vi "ROI entry-Set Z-stack folder path ctrl.vi"(8 "error in (no error)":errorcluster, 11 "Experiment folder path OR Z-stack images folder path":path) -> (0 "error out":errorcluster)   [LabVIEW 2020]
uses:
  ROI Entry screen/Globals/gl_ROI Entry UI globals.vi
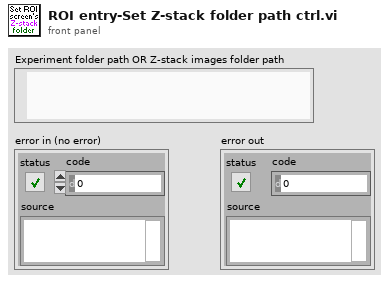
[diagram p1: front panel]
types:
  T1 = typedef "Fixed strings.ctl" = cluster{"ROI file name":string, "Normalised ROI file name":string, "Zplane Pockels values file name":string, "Functional data folder name":string, "Experiment Header file name":string, "Z-stack images folder name":string, "Groups setup rel. path":string, "Groups text file rel. path":string, "TDMS files folder name (F.img)":string, "TDMS files folder name (V.acq)":string, "TDMS files folder name (Pl.acq)":string, "Cycle rel times sequence file":string, "Dynamically called VIs folder name":string, "Time Series folder base name":string}
  T2 = typedef "ROI entry screen ctrl refs cluster.ctl" = cluster{"Done button":refnum<vi>, "Imaging button":refnum<vi>, "Acquisition button":refnum<vi>, "Scan dwell time per pixel (us)":refnum<vi>, "# of planes":refnum<vi>, "Zoom Ctrl":refnum<vi>, "Equal size":refnum<vi>, "Channel":refnum<vi>, "Image Display":refnum<vi>, "Z-Plane Selector":refnum<vi>, "Number of lines left":refnum<vi>, "Z-stack folder path":refnum<vi>, "POI Density":refnum<vi>, "Arb Plane Entry":refnum<vi>, "Whole Plane":refnum<vi>, "Line Mode":refnum<vi>, "Clear Last":refnum<vi>, "Clear All":refnum<vi>, "Delete Lines":refnum<vi>, "Trial Length (sec)":refnum<vi>, "Palette Type":refnum<vi>, "Intensity slider":refnum<vi>, "# POI":refnum<vi>, "Max Z Proj":refnum<vi>, "Zplane ind":refnum<vi>, "Wavelength (nm)":refnum<vi>, "Number of Trials":refnum<vi>, "Funct stim.trig.enable":refnum<vi>, "Funct stim.trig.delay (s)":refnum<vi>, "Line Mode":refnum<vi>, "Step size (µm)":refnum<vi>, "ROI move mode":refnum<vi>, "Cool-down time (s)":refnum<vi>, "Enable cool-down time":refnum<vi>, "Motor Z ind. (um)":refnum<vi>, "AOL Z ind. (um)":refnum<vi>, "Load Reference Image":refnum<vi>, "Rel.  Res.":refnum<vi>, "ROI LIST":refnum<vi>, "Show All":refnum<vi>, "ROI Type":refnum<vi>, "Start Plane":refnum<vi>, "Stop Plane":refnum<vi>, "Offset ROI":refnum<vi>, "Tab Control":refnum<vi>, "Laser Power(%)":refnum<vi>, "Cycle rate":refnum<vi>, "FOV (Ind.)":refnum<vi>, "Frame Size (Ind.)":refnum<vi>, "Resolution (Ind.)":refnum<vi>, "Pixel Density (Ind)":refnum<vi>, "Laser Power (Ind.)":refnum<vi>, "Dwell Time (Ind.)":refnum<vi>, "Adj MC":refnum<vi>}
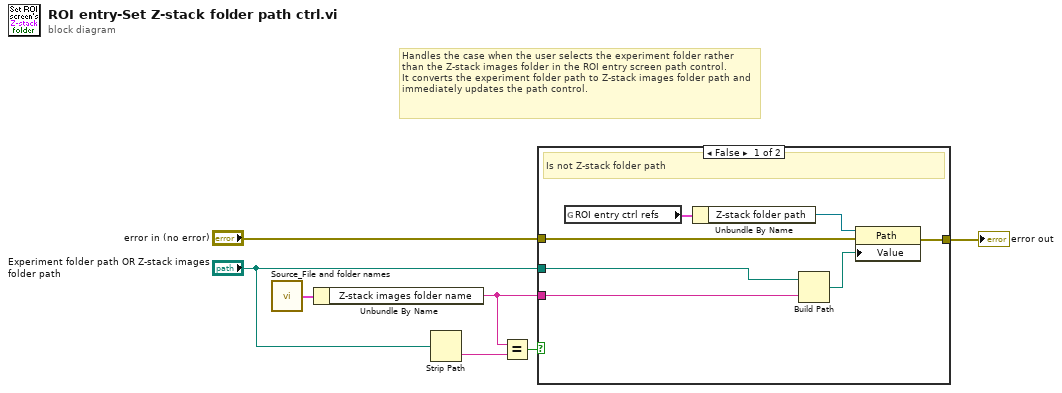
[diagram p0: block diagram]
diagram:
  # "Handles the case when the user selects the experiment folder rather than the Z-stack images folder in the ROI entry screen path control.\nIt converts the experiment folder path to Z-stack images folder path and immediately updates the path control."
  n1 = call "Source_File and folder names.vi"() -> ("Fixed strings"=w4:T1)  [unwired: 1 in]
  n2 = Unbundle By Name(w4) -> ("Z-stack images folder name"=w2:string)
  n3 = Strip Path(path="Experiment folder path OR Z-stack images folder path") -> (name=w5:string)  [unwired: 1 out]
  n4 = Equal?(x=w2, y=w5) -> (x = y?=w1:bool)
  n5 = case shown="False" w1 {
    tunnel: "error in (no error)" -> [w12 w15]
    tunnel: [w11 w15] -> w6
    tunnel: "Experiment folder path OR Z-stack images folder path" -> [w9 _]
    tunnel: w2 -> [w8 _]
    frame False {
      # "Is not Z-stack folder path"
      n6 = global read "gl_ROI Entry UI globals.vi" "ROI entry ctrl refs"() -> (w14:T2)
      n7 = Unbundle By Name(w14) -> ("Z-stack folder path"=w13:refnum<vi>)
      n8 = Build Path(base path=w9, name or relative path=w8) -> (appended path=w10:path)
      n9 = property on="Property Node" class="Path"(reference=w13, error in=w12, "Value"=w10) -> (error out=w11:errorcluster)  [unwired: 1 out]
    }
    frame True {
      # "Is Z-stack folder path"
    }
  }
  "error out" <- w6
